vi "calculate.vi"(11 "Formular":string) -> (2 "Value":dbl, 3 "Result":string)   [LabVIEW 2020]
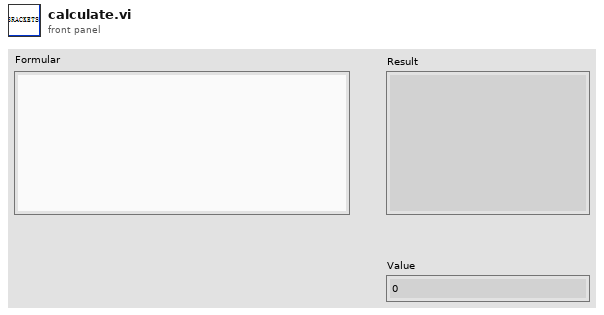
[diagram p1: front panel]
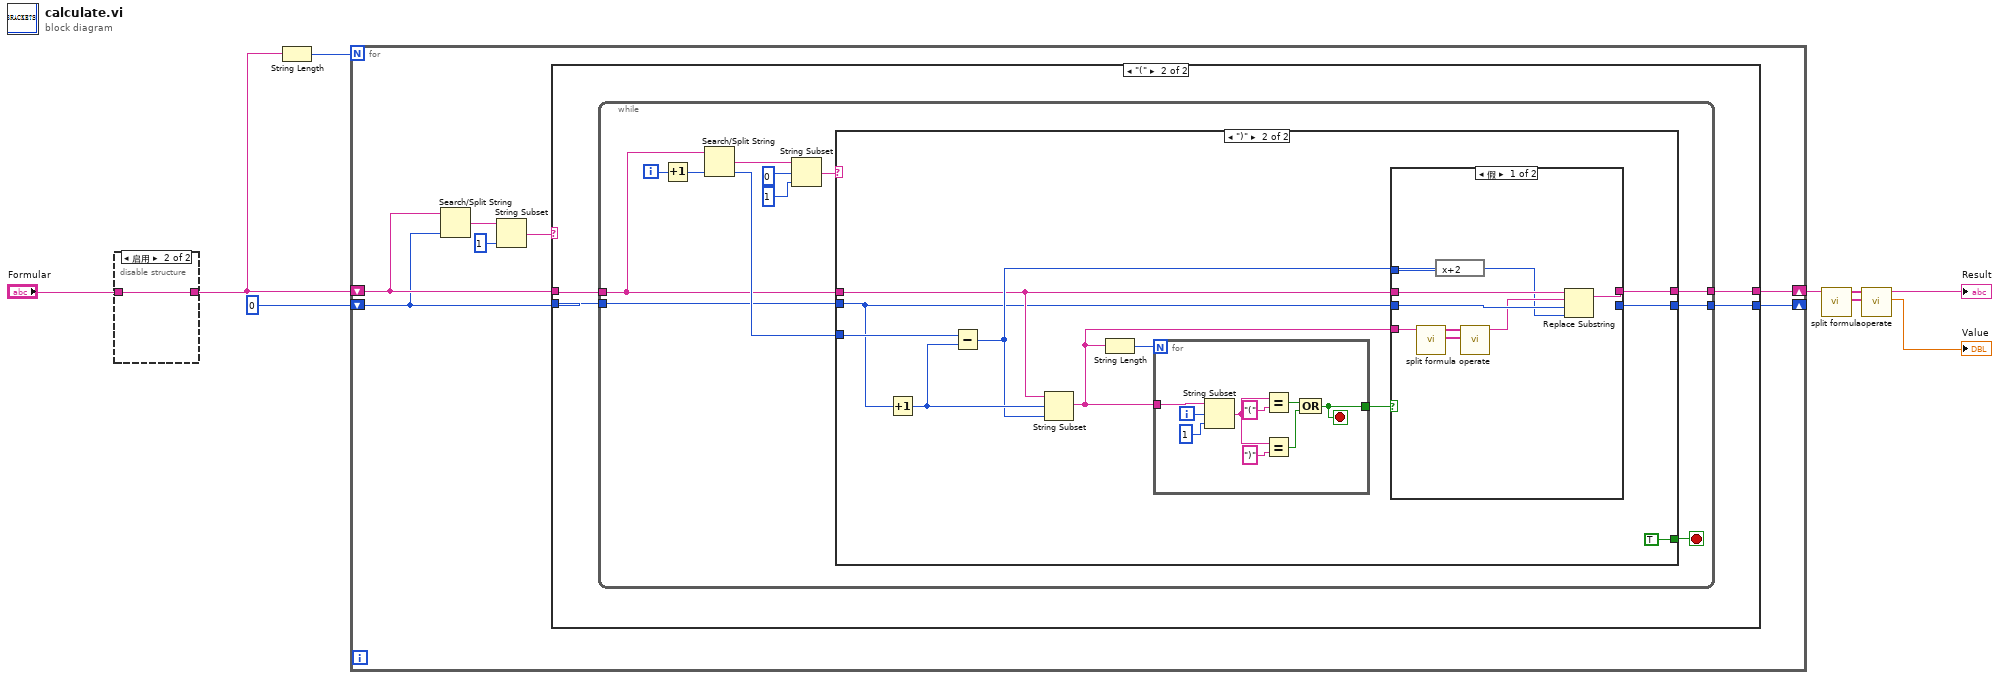
[diagram p0: block diagram]
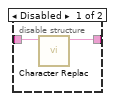
[diagram p2: hidden frame]
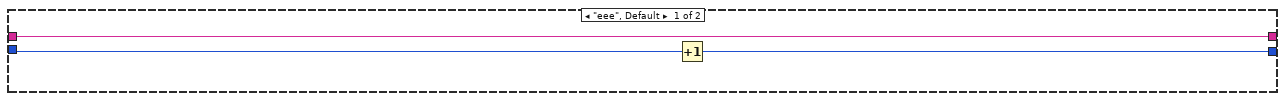
[diagram p3: hidden frame]
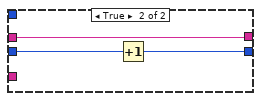
[diagram p5: hidden frame]
diagram:
  n1 = disable-structure shown="启用" {
    disable-tunnel: "Formular" -> [w11 w12]
    disable-tunnel: [w10 w12] -> w2
    frame Disabled {
      n2 = call "Character Replac.vi"("字符串"=w11) -> ("连接的字符串"=w10:string)  [unwired: 10 in]
    }
    frame Enabled {
    }
  }
  n3 = String Length(string=w2) -> (length=w8:i32)
  n4 = for {
    N: w8 -> [_]
    shift-right: [w18] -> w7
    shift-left: w2 -> [w19]
    shift-right: [w17] -> _
    shift-left: 0 -> [w14]
    n5 = Search/Split String(string=w19, offset (0)=w14) -> (match + rest of string=w16:string)  [unwired: 1 in, 2 out]
    n6 = String Subset(string=w16, length (rest)=1 ("长度（剩余）")) -> (substring=w13:string)  [unwired: 1 in]
    n7 = case shown="\"(\"" w13 {
      tunnel: w19 -> [w20 w26]
      tunnel: w14 -> [w22 w25]
      tunnel: [w20 w24] -> w18
      tunnel: [w21 w23] -> w17
      frame "eee", Default {
        n8 = Increment(x=w22) -> (x+1=w21:i32)
      }
      frame "(" {
        n9 = while {
          tunnel: w26 -> [w29]
          tunnel: w25 -> [w28]
          tunnel: [w32] -> w24
          tunnel: [w30] -> w23
          i -> [w38]
          stop <- w31 stop-if-true
          n10 = Increment(x=w38) -> (x+1=w37:i32)
          n11 = Search/Split String(string=w29, offset (0)=w37) -> (match + rest of string=w36:string, offset of match=w33:i32)  [unwired: 1 in, 1 out]
          n12 = String Subset(string=w36, offset (0)=0 ("偏移量(0)"), length (rest)=1 ("长度（剩余）")) -> (substring=w27:string)
          n13 = case shown="\")\"" w27 {
            tunnel: w29 -> [_ w43]
            tunnel: w33 -> [_ w49]
            tunnel: w28 -> [_ w42]
            tunnel: [_ w48] -> w32
            tunnel: [_ TRUE] -> w31
            tunnel: [_ w44] -> w30
            frame "eee", Default {
            }
            frame ")" {
              n14 = Increment(x=w42) -> (x+1=w47:i32)
              n15 = Subtract(x=w49, y=w47) -> (x-y=w46:i32)
              n16 = String Subset(string=w43, offset (0)=w47, length (rest)=w46) -> (substring=w40:string)
              n17 = String Length(string=w40) -> (length=w39:i32)
              n18 = for {
                N: w39 -> [_]
                tunnel: w40 -> [w58]
                tunnel: [w50] -> w45
                i -> [w51]
                stop <- w50 stop-if-true
                n19 = String Subset(string=w58, offset (0)=w51, length (rest)=1 ("长度（剩余）")) -> (substring=w54:string)
                n20 = Equal?(x=w54, y="(") -> (x = y?=w53:bool)
                n21 = Equal?(x=w54, y=")") -> (x = y?=w52:bool)
                n22 = Compound Arithmetic op=OR(w53, w52) -> (w50:bool)
              }
              n23 = case shown="假" w45 {
                tunnel: w40 -> [w63 _]
                tunnel: w42 -> [w67 w69]
                tunnel: [w66 w70] -> w48
                tunnel: w46 -> [w64 _]
                tunnel: w43 -> [w60 w70]
                tunnel: [_ w68] -> w44
                frame False {
                  n24 = call "split formula.vi"("Formula"=w63) -> ("Symbol"=w62:string[], "Element"=w61:string[])  [unwired: 9 in]
                  n25 = expression code="x+2"(w64) -> (w59:i32)
                  n26 = call "operate.vi"("symbol"=w62, "Element"=w61) -> ("Result"=w65:string)  [unwired: 8 in, 1 out]
                  n27 = Replace Substring(2:w59, 3:w67, 4:w65, 5:w60) -> (1:w66:string)  [unwired: 1 out]
                }
                frame True {
                  n28 = Increment(x=w69) -> (x+1=w68:i32)
                }
              }
            }
          }
        }
      }
    }
  }
  n29 = call "split formula.vi"("Formula"=w7) -> ("Symbol"=w5:string[], "Element"=w6:string[])  [unwired: 9 in]
  n30 = call "operate.vi"("symbol"=w5, "Element"=w6) -> ("Value"=→"Value":dbl, "Result"=→"Result":string)  [unwired: 8 in]
